vi "DAQmx.Write.vi"(8 "error in (no error)":errorcluster, 10 "AOwfm":waveform(dbl)[](array[waveform]), 11 "DAQmx in":refnum<class "DAQmx.lvclass">) -> (0 "error out":errorcluster, 3 "DAQmx out":refnum<class "DAQmx.lvclass">, 4 "AO time (s)":dbl=53.0 format="%#_6p")   [LabVIEW 2019, in "DAQmx.lvclass"]
uses:
  DAQmx.lvclass
  DAQmx.lvclass/DAQmx.ctl
  <vilib>/DAQmx/write.llb/DAQmx Write (Analog 1D Wfm NChan NSamp).vi
  <vilib>/DAQmx/miscellaneous.llb/DAQmx Fill In Error Info.vi
panel:
  out "Number of Samples written per channel":u32[](array[numeric])
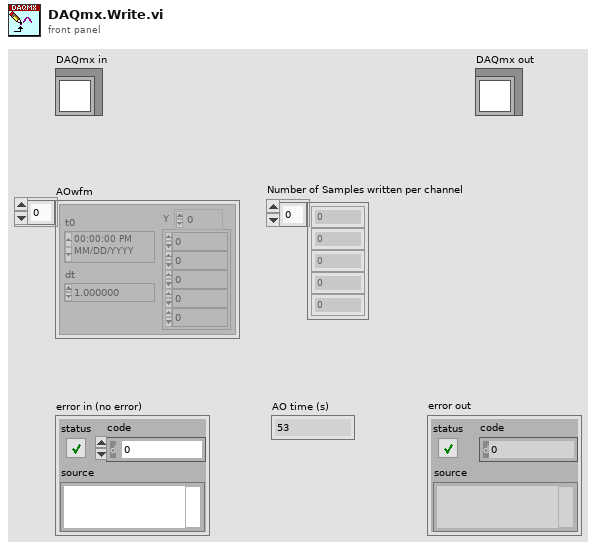
[diagram p1: front panel]
types:
  T1 = typedef "DAQmx.lvclass/DAQmx.Channel Map--Cluster.ctl" = cluster{"task":refnum<k21>, "Device":tag, "Offset":u32, "Count":u32, "DevIsSimulated":bool}
  T2 = cluster{"task":refnum<k21>, "Array":waveform(dbl)[]}[]
  T3 = cluster{"task":refnum<k21>, "Array":waveform(dbl)[]}
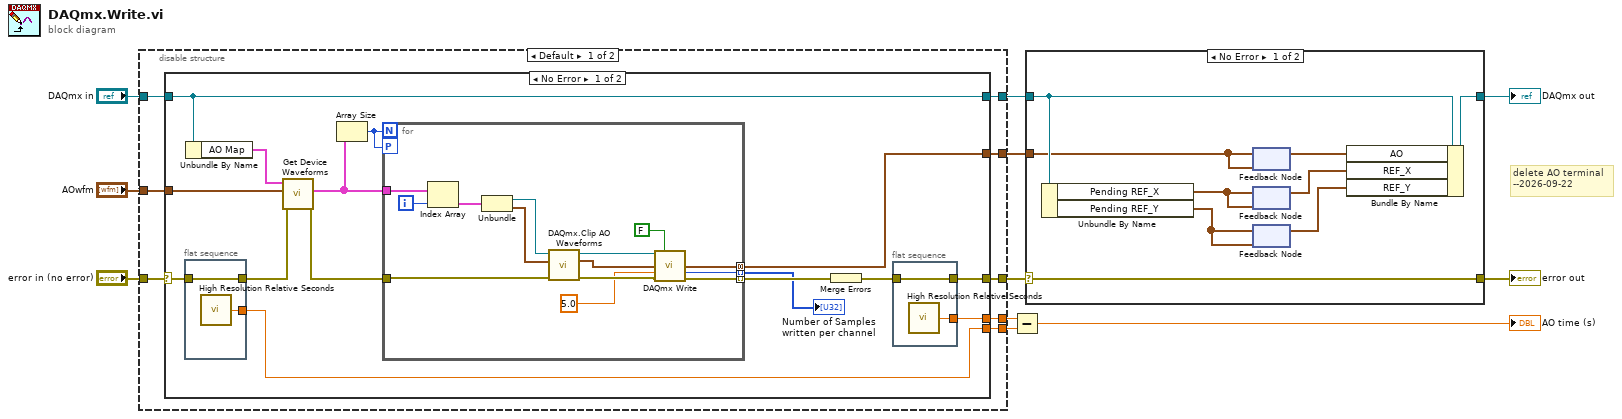
[diagram p0: block diagram]
diagram:
  # "delete AO terminal\n--2026-09-22"
  n1 = disable-structure shown="Default" {
    disable-tunnel: [w19 w55] -> w2
    disable-tunnel: "DAQmx in" -> [w17 w54]
    disable-tunnel: "AOwfm" -> [w18 _]
    disable-tunnel: "error in (no error)" -> [w13 w55]
    disable-tunnel: [w16 w54] -> w1
    disable-tunnel: [w15 _] -> w11
    disable-tunnel: [w14 _] -> w8
    disable-tunnel: [w12 _] -> w5
    frame condition #0 (active) {
      n2 = case shown="No Error" w13 {
        selector: w13 -> [w31 w52]
        tunnel: [w33 w52] -> w19
        tunnel: w18 -> [w22 _]
        tunnel: w17 -> [w21 w53]
        tunnel: [w21 w53] -> w16
        tunnel: [w32 _] -> w15
        tunnel: [w30 _] -> w14
        tunnel: [w27 _] -> w12
        frame No Error {
          n3 = flat-sequence {
            tunnel: w31 -> [w37]
            tunnel: [w37] -> w23
            tunnel: [w38] -> w30
            frame #0 {
              n4 = call <vilib>:"High Resolution Relative Seconds.vi"() -> ("relative seconds"=w38:dbl)
            }
          }
          n5 = Unbundle By Name(w21) -> ("AO Map"=w20:T1[])
          n6 = call "Get Device Waveforms.vi"("error in (no error)"=w23, "AOwfm"=w22, "Channel Map"=w20) -> ("error out"=w26:errorcluster, "Device Waveforms"=w24:T2)  [unwired: 7 in]
          n7 = Array Size(array=w24) -> (size(s)=w25:i32)
          n8 = for {
            N: w25 -> [_]
            tunnel: w24 -> [w51]
            tunnel: w26 -> [w44]
            tunnel: [w50] -> w34 mode=indexing
            workers-P: w25 -> [_]
            tunnel: [w49] -> w28 mode=indexing
            tunnel: [w45] -> w27 mode=concatenating
            i -> [w47]
            n9 = Index Array(array=w51, index=w47) -> (element=w41:T3)
            n10 = Unbundle(w41) -> ("task"=w39:refnum<k21>, "Array"=w40:waveform(dbl)[])
            n11 = call "DAQmx.Clip AO Waveforms.vi"("error in (no error)"=w44, "AO []"=w40, "task"=w39) -> ("error out"=w43:errorcluster, "Clipped AO []"=w45:waveform(dbl)[], "task out"=w46:refnum<k21>)  [unwired: 6 in]
            n12 = call-poly <vilib>:"DAQmx Write.vi"("task/channels in"=w46, "auto start"=FALSE, "data"=w45, "timeout"=5.0, "error in"=w43) -> ("number of samples written per channel"=w49:u32, "error out"=w50:errorcluster)  [unwired: 8 in, 1 out]
          }
          "Number of Samples written per channel" <- w28
          n13 = Merge Errors(w34) -> (w29:errorcluster)
          n14 = flat-sequence {
            tunnel: w29 -> [w35]
            tunnel: [w35] -> w33
            tunnel: [w36] -> w32
            frame #0 {
              n15 = call <vilib>:"High Resolution Relative Seconds.vi"() -> ("relative seconds"=w36:dbl)
            }
          }
        }
        frame Error {
        }
      }
    }
    frame condition #1 {
    }
  }
  n16 = Subtract(x=w11, y=w8) -> (x-y=→"AO time (s)":dbl)
  n17 = case shown="No Error" w2 {
    selector: w2 -> [w58 w65]
    tunnel: w5 -> [w56 _]
    tunnel: w1 -> [w63 w66]
    tunnel: [w59 w66] -> w4
    tunnel: [w58 w65] -> w3
    frame No Error {
      n18 = Unbundle By Name(w63) -> ("Pending REF_X"=w64:waveform(dbl)[], "Pending REF_Y"=w57:waveform(dbl)[])
      n19 = feedback #1(w56) -> (w62:waveform(dbl)[])
      n20 = feedback-in #1(w56) -> ()
      n21 = feedback #2(w64) -> (w61:waveform(dbl)[])
      n22 = feedback-in #2(w64) -> ()
      n23 = feedback #3(w57) -> (w60:waveform(dbl)[])
      n24 = feedback-in #3(w57) -> ()
      n25 = Bundle By Name(cluster=w63, "AO"=w62, "REF_X"=w61, "REF_Y"=w60) -> (w59:refnum<class "DAQmx.lvclass">)
    }
    frame Error {
    }
  }
  "error out" <- w3
  "DAQmx out" <- w4
